vi "LIA Filter and Decimate Continuous.vi"(7 "Boolean":bool, 11 "Array":dbl[](array[numeric])) -> (3 "Decimated Array":dbl[](array[numeric]))   [LabVIEW 2017]
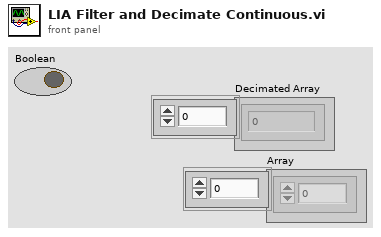
[diagram p1: front panel]
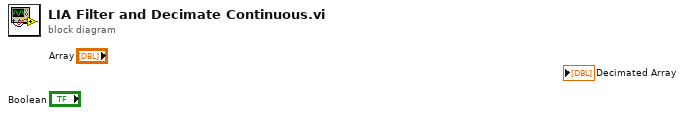
[diagram p0: block diagram]
diagram:
